vi "Leap.vi"() -> ()   [LabVIEW 2017]
uses:
  <vilib>/MakerHub/Leap/Private/Type Defs/Swipe Direction.ctl
  <vilib>/MakerHub/Leap/Public/Gestures/Swipe/Instance VIs/Read 1 Swipe Direction.vi
  <vilib>/MakerHub/Leap/LMH-Leap.lvlib
panel:
  out "Boolean 4":bool
  out "Boolean 3":bool
  out "NewVal":T1
  in  "Swipe Direction":T1
  out "Boolean 2":bool
  in  "stop":bool
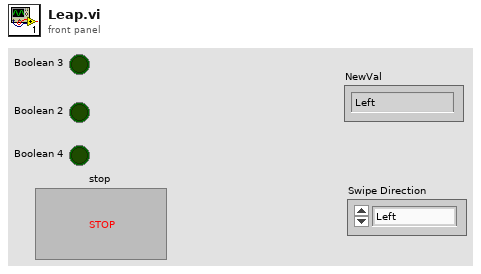
[diagram p1: front panel]
types:
  T1 = typedef "LMH-Leap.lvlib/Swipe Direction.ctl" = enum16{"Left", "Right", "Up", "Down", "In", "Out"}
  T2 = typedef "LMH-Leap.lvlib/Leap Handle.ctl" = cluster{"LeapCSharp":refnum<k24>}
  T3 = typedef "LMH-Leap.lvlib/Gesture State.ctl" = enum16{"Invalid", "Start", "Update", "Stop"}
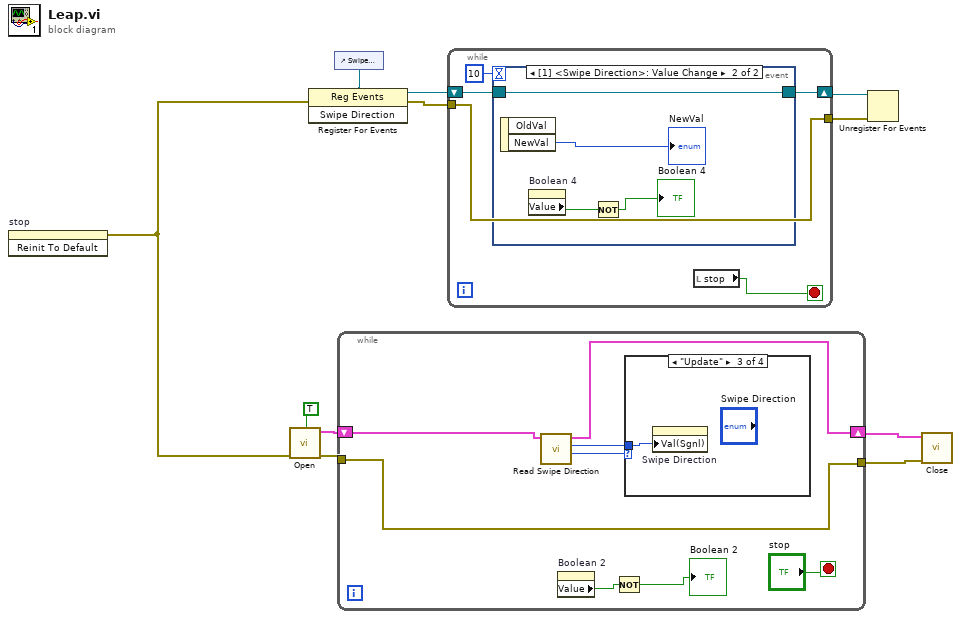
[diagram p0: block diagram]
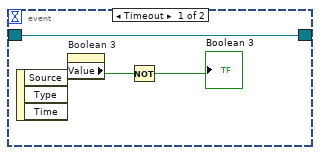
[diagram p2: hidden frame]
diagram:
  n1 = invoke on="stop" class="Bool (strict)" method="Reinit To Default"() -> (error out=w1:errorcluster)  [unwired: 3 in, 2 out]
  n2 = call <vilib>:"Open.vi"("Error In"=w1, "Enable Gestures? (T)"=TRUE) -> ("Error Out"=w4:errorcluster, "Leap Handle"=w8:T2)  [unwired: 8 in]
  n3 = control-ref of="Swipe Direction"() -> (w9:refnum<vi>)
  n4 = register-events(error in=w1, w9) -> (reference out=w7:refnum<event-registration>, error out=w5:errorcluster)  [unwired: 1 in]
  n5 = while {
    tunnel: [w18] -> w2
    tunnel: w4 -> [w18]
    shift-right: [w19] -> w10
    shift-left: w8 -> [w12]
    stop <- "stop" stop-if-true
    n6 = call-poly <vilib>:"Read Swipe Direction.vi"("Leap Handle"=w12) -> ("Gesture State"=w15:T3, "Swipe Direction"=w14:T1, "Leap Handle"=w19:T2)  [unwired: 7 in, 1 out]
    n7 = property on="Boolean 2" class="Bool (strict)"() -> ("Value"=w17:bool)  [unwired: 2 in, 2 out]
    n8 = Not(x=w17) -> (.not. x?=→"Boolean 2":bool)
    n9 = case shown="\"Update\"" w15 {
      tunnel: w14 -> [_ _ w20 _]
      frame "Invalid", Default {
      }
      frame "Start" {
      }
      frame "Update" {
        n10 = property on="Swipe Direction" class="Enum (strict)"("Val(Sgnl)"=w20) -> ()  [unwired: 2 in, 2 out]
      }
      frame "Stop" {
      }
    }
  }
  n11 = while {
    shift-right: [w24] -> w6
    shift-left: w7 -> [w25]
    tunnel: w5 -> [w22]
    tunnel: [w22] -> w3
    stop <- w21 stop-if-true
    n12 = event shown="[1] <Swipe Direction>: Value Change" {
      selector: w25 -> [w26 w31]
      dyn-events: [w26 w31] -> w24
      timeout: 10 -> [_ _]
      event Timeout {
        n13 = event-data() -> ()  [unwired: 1 in, 3 out]
        n14 = property on="Boolean 3" class="Bool (strict)"() -> ("Value"=w28:bool)  [unwired: 2 in, 2 out]
        n15 = Not(x=w28) -> (.not. x?=→"Boolean 3":bool)
      }
      event Value Change {
        n16 = event-data() -> ("NewVal"=→"NewVal":T1)  [unwired: 1 in, 1 out]
        n17 = property on="Boolean 4" class="Bool (strict)"() -> ("Value"=w30:bool)  [unwired: 2 in, 2 out]
        n18 = Not(x=w30) -> (.not. x?=→"Boolean 4":bool)
      }
    }
    n19 = local read "stop"() -> (w21:bool)
  }
  n20 = Unregister For Events(event registration refnum=w6, error in=w3) -> ()  [unwired: 1 out]
  n21 = call <vilib>:"Close.vi"("Error In"=w2, "Leap Handle"=w10) -> ()  [unwired: 9 in, 1 out]
